vi "TilePlot.vi"(0 "Array":dbl[][](array[numeric])=array100x100[10000 elements] format="%.2f", 1 "Height (pixels)":dbl=350.0, 2 "Width (pixels)":dbl=400.0, 3 "DPI":dbl=63.0, 4 "Left":dbl=0.06 format="%#_13g", 5 "Right":dbl=0.06 format="%#_13g", 6 "Max":dbl, 7 "Bottom":dbl=0.12 format="%#_13g", 8 "Min":dbl, 9 "Top":dbl=0.03 format="%#_13g") -> (14 "Tile Plot":picture, 17 "Max":dbl)   [LabVIEW 2014]
uses:
  <vilib>/Heliosphere Research LLC/Advanced Plotting Toolkit/properties/Colormap_Map.ctl
  <vilib>/Heliosphere Research LLC/Advanced Plotting Toolkit/typedefs/PlotColor.ctl
  <vilib>/Heliosphere Research LLC/Advanced Plotting Toolkit/api_plotting/TilesProperties.ctl
  <vilib>/Heliosphere Research LLC/Advanced Plotting Toolkit/properties/Colormap.ctl
  <vilib>/Heliosphere Research LLC/Advanced Plotting Toolkit/properties/Colormap_Scaling.ctl
  <vilib>/Heliosphere Research LLC/Advanced Plotting Toolkit/properties/Line.ctl
  <vilib>/Heliosphere Research LLC/Advanced Plotting Toolkit/properties/Line_Style.ctl
  <vilib>/Heliosphere Research LLC/Advanced Plotting Toolkit/properties/Display.ctl
  <vilib>/Heliosphere Research LLC/Advanced Plotting Toolkit/api_core/NewPlotProperties.ctl
  <vilib>/Heliosphere Research LLC/Advanced Plotting Toolkit/Advanced Plotting Toolkit.lvlib
panel:
  in  "?":enum32{"Settings", "Plot", "Data"}(tab)
  in  "Reverse":bool
  in  "Label":string
  in  "Colormap":T1=enum."Hot and Cold"
  in  "Line Width":sgl=nan
  in  "Line Color":T2=2147483647 items=["Automatic"=2147483647, "Black"=0, "White"=16777215, "Red"=16711680, "Green"=2263842, "Blue"=255, "Cyan"=65535, "Magenta"=16711935, "Yellow"=16776960]
  in  "Axis Background":T2=2147483647 items=["Automatic"=2147483647, "Black"=0, "White"=16777215, "Red"=16711680, "Green"=2263842, "Blue"=255, "Cyan"=65535, "Magenta"=16711935, "Yellow"=16776960]
  in  "Background Color":T2=2147483647 items=["Automatic"=2147483647, "Black"=0, "White"=16777215, "Red"=16711680, "Green"=2263842, "Blue"=255, "Cyan"=65535, "Magenta"=16711935, "Yellow"=16776960]
  in  "Ratio":dbl=nan format="%#_13g"
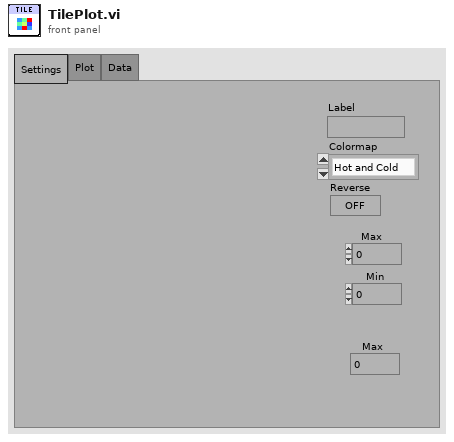
[diagram p1: front panel]
types:
  T1 = typedef "Advanced Plotting Toolkit.lvlib/Colormap_Map.ctl" = enum16{"Automatic", "Rainbow", "Hot and Cold", "White-Black", "White-Blue", "White-Green", "White-Red", "Fire", "Water", "Earth", "Air", "Pastel", "Banded", "Stepped"}
  T2 = typedef "Advanced Plotting Toolkit.lvlib/PlotColor.ctl" = u32
  T3 = typedef "Advanced Plotting Toolkit.lvlib/NewPlotProperties.ctl" = cluster{"Background Color":T2, "Axis Background":T2, "Left Margin":dbl, "Right Margin":dbl, "Bottom Margin":dbl, "Top Margin":dbl, "Aspect Ratio":dbl}
  T4 = typedef "Advanced Plotting Toolkit.lvlib/TilesProperties.ctl" = cluster{"Colormap":T5, "Line":T7, "Display":T9}
  T5 = typedef "Advanced Plotting Toolkit.lvlib/Colormap.ctl" = cluster{"Map":T1, "Value Min":dbl, "Value Max":dbl, "Scaling":T6, "Reverse":bool}
  T6 = typedef "Advanced Plotting Toolkit.lvlib/Colormap_Scaling.ctl" = enum16{"Default"}
  T7 = typedef "Advanced Plotting Toolkit.lvlib/Line.ctl" = cluster{"Style":T8, "Color":T2, "Width":sgl}
  T8 = typedef "Advanced Plotting Toolkit.lvlib/Line_Style.ctl" = enum16{"Automatic", "Solid", "Dashed", "Dotted", "Dash-dot", "Invisible"}
  T9 = typedef "Advanced Plotting Toolkit.lvlib/Display.ctl" = cluster{"Alpha":dbl, "Z Order":dbl}
  T10 = typedef "Advanced Plotting Toolkit.lvlib/PlotID.ctl" = i32
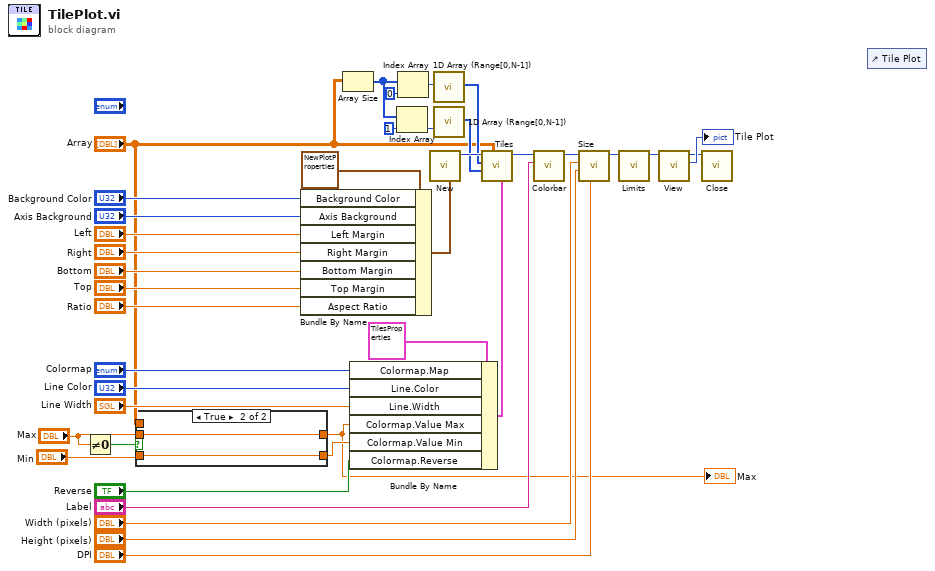
[diagram p0: block diagram]
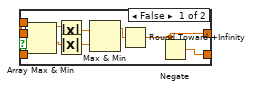
[diagram p2: hidden frame]
diagram:
  n1 = Not Equal To 0?(x="Max") -> (x != 0?=w5:bool)
  n2 = case shown="True" w5 {
    tunnel: [w40 w49] -> w2
    tunnel: "Array" -> [w42 _]
    tunnel: "Max" -> [_ w49]
    tunnel: [w41 w48] -> w4
    tunnel: "Min" -> [_ w48]
    frame False {
      n3 = Array Max & Min(array=w42) -> (max value=w46:dbl, min value=w47:dbl)  [unwired: 2 out]
      n4 = Absolute Value(x=w46) -> (abs(x)=w45:dbl)
      n5 = Absolute Value(x=w47) -> (abs(x)=w44:dbl)
      n6 = Max & Min(x=w45, y=w44) -> (max(x,y)=w43:dbl)  [unwired: 1 out]
      n7 = Round Toward +Infinity(x=w43) -> (ceil(x): smallest int >= x=w40:dbl)
      n8 = Negate(x=w40) -> (-x=w41:dbl)
    }
    frame True {
    }
  }
  "Max" <- w2
  n9 = Bundle By Name(cluster=T3 {"Background Color"=2147483647, "Axis Background"=2147483647, "Left Margin"=0.05, "Right Margin"=0.15, "Bottom Margin"=0.03, "Top Margin"=0.03, "Aspect Ratio"=nan} ("New Plot Properties"), "Background Color"="Background Color", "Axis Background"="Axis Background", "Left Margin"="Left", "Right Margin"="Right", "Bottom Margin"="Bottom", "Top Margin"="Top", "Aspect Ratio"="Ratio") -> (w8:T3)
  n10 = Array Size(array="Array") -> (size(s)=w28:i32[])
  n11 = Bundle By Name(cluster=T4 {"Colormap"={"Map"=enum."Automatic", "Value Min"=nan, "Value Max"=nan, "Scaling"=enum."Default", "Reverse"=FALSE}, "Line"={"Style"=enum."Automatic", "Color"=2147483647, "Width"=nan}, "Display"={"Alpha"=nan, "Z Order"=nan}} ("Properties"), "Colormap.Map"="Colormap", "Line.Color"="Line Color", "Line.Width"="Line Width", "Colormap.Value Max"=w2, "Colormap.Value Min"=w4, "Colormap.Reverse"="Reverse") -> (w16:T4)
  n12 = Index Array(array=w28, index=1) -> (element=w26:i32)
  n13 = Index Array(array=w28, index=0) -> (element=w27:i32)
  n14 = call <vilib>:"New.vi"("Properties"=w8) -> ("Plot ID"=w37:T10)  [unwired: 9 in, 1 out]
  n15 = call "1D Array (Range[0,N-1]).vi"("Range"=w27) -> ("Array"=w24:i32[])  [unwired: 18 in]
  n16 = call "1D Array (Range[0,N-1]).vi"("Range"=w26) -> ("Array"=w25:i32[])  [unwired: 18 in]
  n17 = call <vilib>:"Tiles.vi"("Properties"=w16, "Z Data"="Array", "Y Tile Boundaries"=w25, "X Tile Boundaries"=w24, "Plot ID"=w37) -> ("Plot ID Out"=w34:T10)  [unwired: 5 in, 1 out]
  n18 = call <vilib>:"Colorbar.vi"("Label"="Label", "Plot ID"=w34) -> ("Plot ID Out"=w23:T10)  [unwired: 8 in, 1 out]
  n19 = call <vilib>:"Size.vi"("DPI"="DPI", "Height (pixels)"="Height (pixels)", "Width (pixels)"="Width (pixels)", "Plot ID"=w23) -> ("Plot ID Out"=w18:T10)  [unwired: 6 in, 1 out]
  n20 = call <vilib>:"Limits.vi"("Plot ID"=w18) -> ("Plot ID Out"=w19:T10)  [unwired: 9 in, 1 out]
  n21 = call <vilib>:"View.vi"("Plot ID"=w19) -> ("Picture"=→"Tile Plot":picture, "Plot ID Out"=w38:T10)  [unwired: 8 in, 1 out]
  n22 = call <vilib>:"Close.vi"("Plot ID"=w38) -> ()  [unwired: 10 in, 1 out]
  n23 = control-ref of="Tile Plot"() -> ()  [unwired: 1 out]
